vi "Agilent PWM Read Calibration Status.vi"(7 "Agilent PWM":T1, 8 "error in (no error)":errorcluster, 11 "VISA Resource Name":refnum<visa-resource-name>) -> (0 "error out":errorcluster {"code" format="%.0x"}, 2 "Calibrated?":bool, 3 "dup VISA Resource Name":refnum<visa-resource-name>)   [LabVIEW 2011]
uses:
  TypeDefs/Agilent PWM Instrument Info.ctl
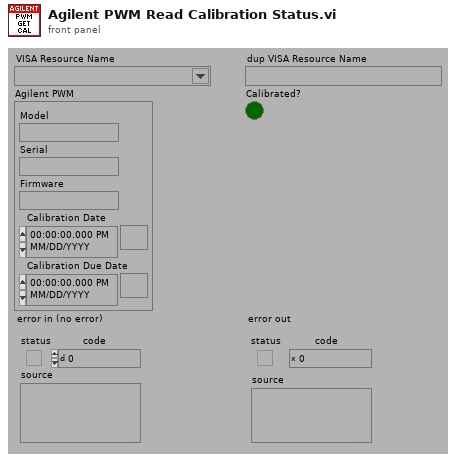
[diagram p1: front panel]
types:
  T1 = typedef "Agilent PWM Instrument Info.ctl" = cluster{"Model":string, "Serial":string, "Firmware":string, "Calibration Date":timestamp, "Calibration Due Date":timestamp}
  T2 = typedef "Agilent PWM Model.ctl" = enum16{"Not Supported", "E4418X", "E4419X", "U2000X"}
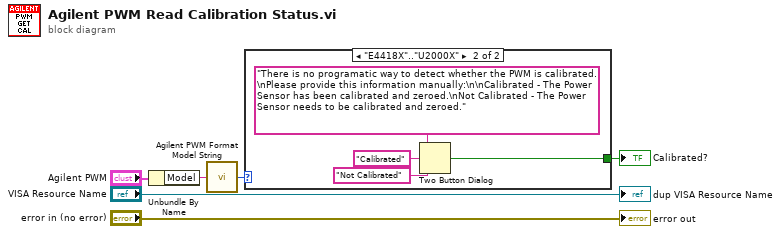
[diagram p0: block diagram]
diagram:
  n1 = Unbundle By Name("Agilent PWM") -> ("Model"=w3:string)
  n2 = call "Agilent PWM Format Model String.vi"("Model"=w3) -> ("Model"=w1:T2)
  n3 = case shown="\"E4418X\"..\"U2000X\"" w1 {
    tunnel: [_ w9] -> w4
    frame "Not Supported" {
    }
    frame "E4418X".."U2000X" {
      n4 = Two Button Dialog(message="There is no programatic way to detect whether the PWM is calibrated.\nPlease provide this information manually:\n\nCalibrated - The Power Sensor has been calibrated and zeroed.\nNot Calibrated - The Power Sensor needs to be calibrated and zeroed.", 1:"Not Calibrated" ("T button name (\"OK\")"), 2:"Calibrated" ("T button name (\"OK\")")) -> (T button?=w9:bool)
    }
  }
  "Calibrated?" <- w4
  "error out" <- "error in (no error)"
  "dup VISA Resource Name" <- "VISA Resource Name"
